vi "Simple TCP - Client.vi"() -> ()   [LabVIEW 2020]
doc: "Demonstrates how to open a connection to an TCP server, read the data being sent, and display the data on a chart. This VI is designed to stop if the TCP connection is terminated."
panel:
  out "Color Box":u32(colorbox)
  in  "Test Mode:":string(combo)
  in  "Stop":bool
  out "Status":string
  in  "Start":bool
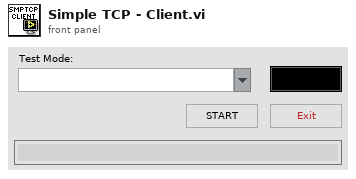
[diagram p1: front panel]
types:
  T1 = enum32{"Invalid", "Standard", "Closed", "Hidden", "Minimized", "Maximized"}
  T2 = enum32{"invalid app kind", "Development System", "Run Time System", "Student Edition", "Embedded LabVIEW", "Evaluation", "Custom"}
  T3 = cluster{"Core":cluster{"Current VI Reference":refnum<vi>, "Close Panel on Exit?":bool}, "Your Boolean data":bool, "IP Address":string, "port":u16, "connection ID":refnum<k5>, "Status":string, "Command":string, "Response":string}
  T4 = cluster{"Current VI Reference":refnum<vi>, "Close Panel on Exit?":bool}
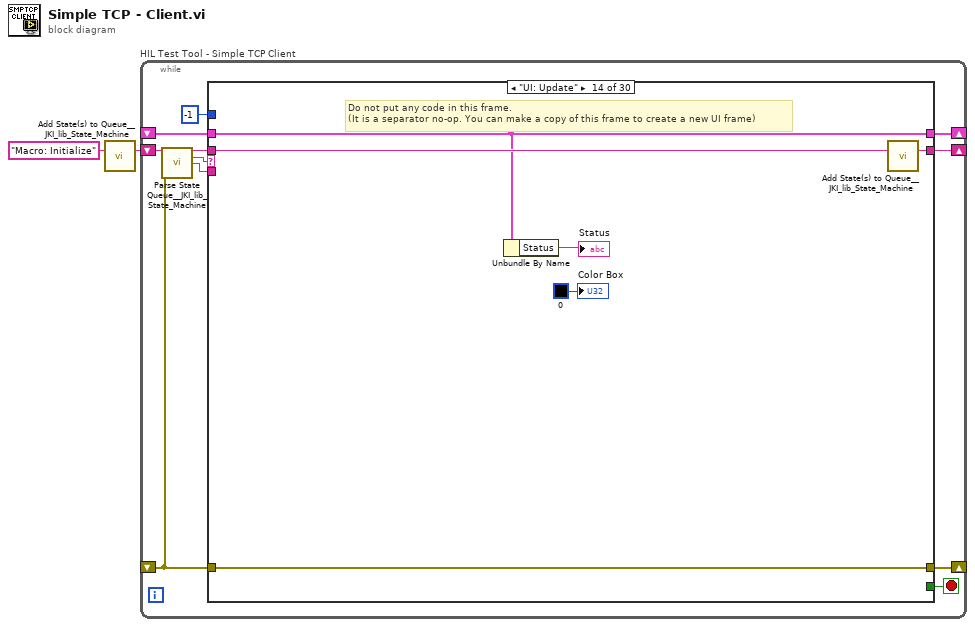
[diagram p0: block diagram]
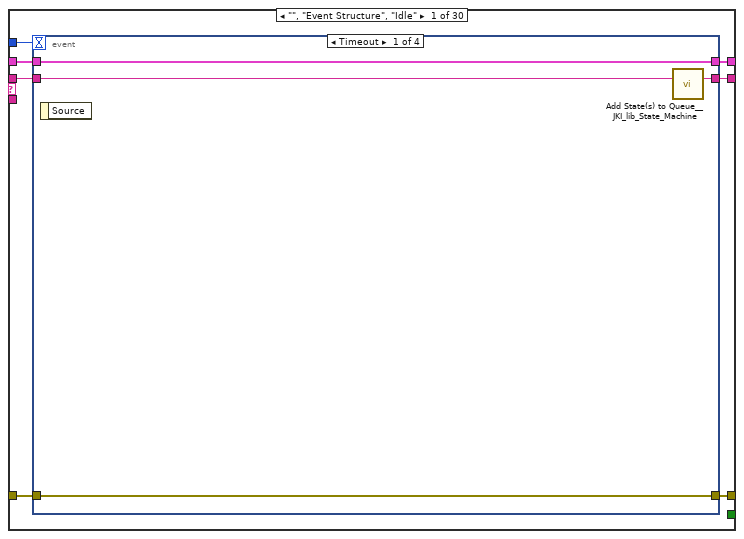
[diagram p2: hidden frame]
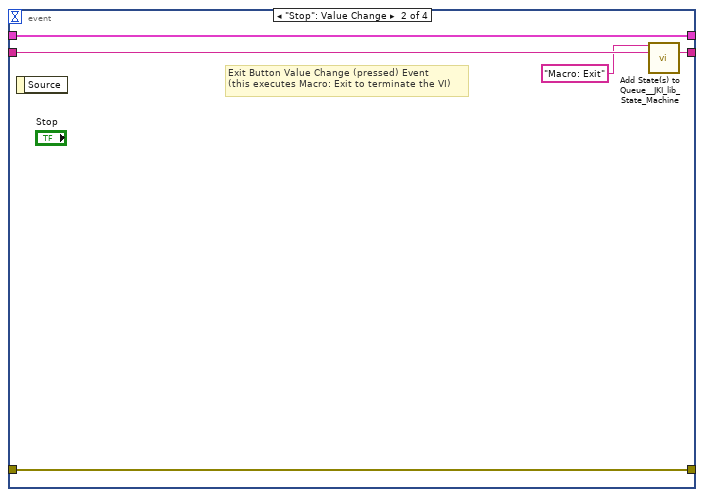
[diagram p3: hidden frame]
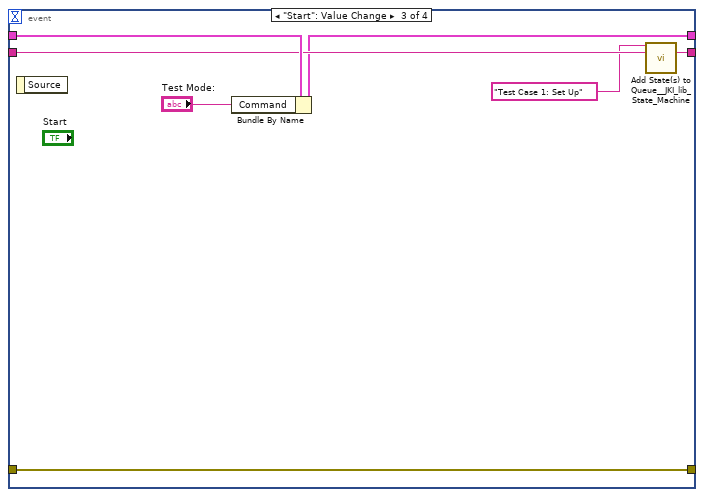
[diagram p4: hidden frame]
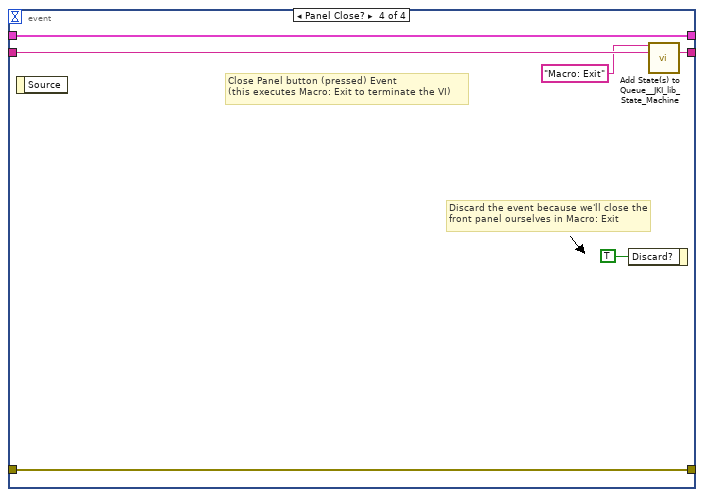
[diagram p5: hidden frame]
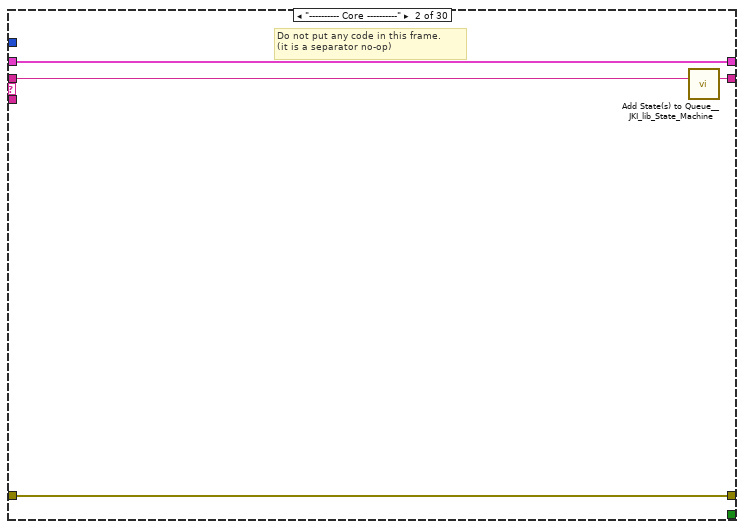
[diagram p6: hidden frame]
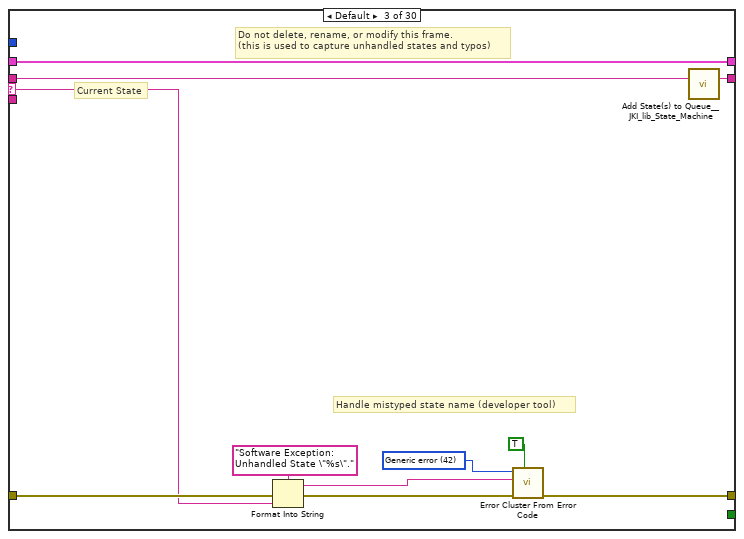
[diagram p7: hidden frame]
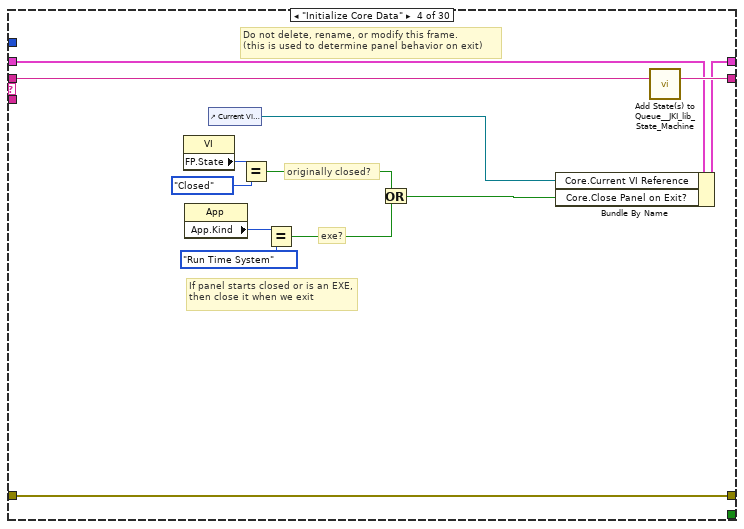
[diagram p8: hidden frame]
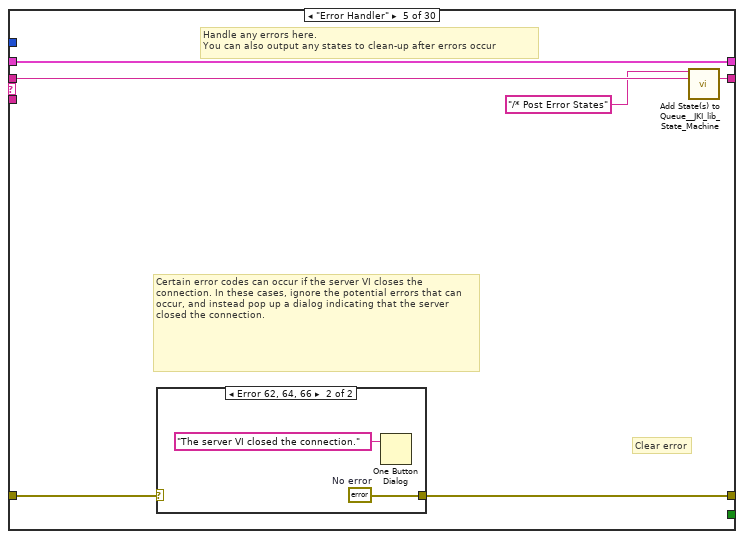
[diagram p9: hidden frame]
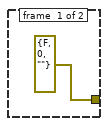
[diagram p10: hidden frame]
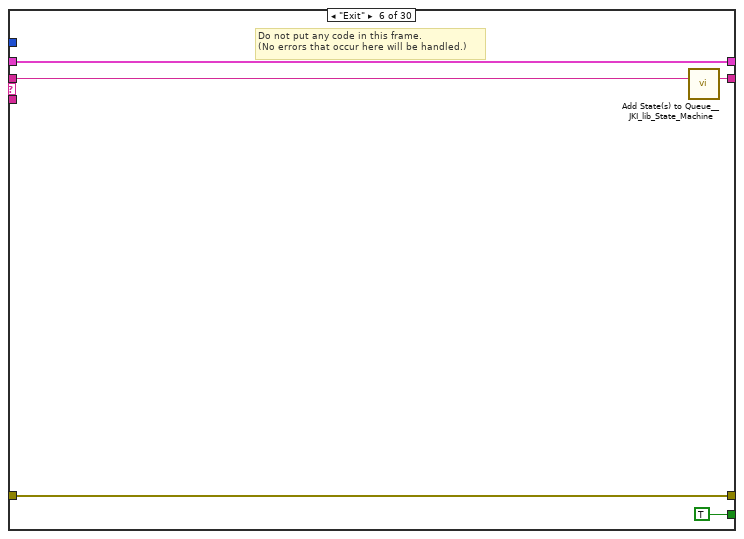
[diagram p11: hidden frame]
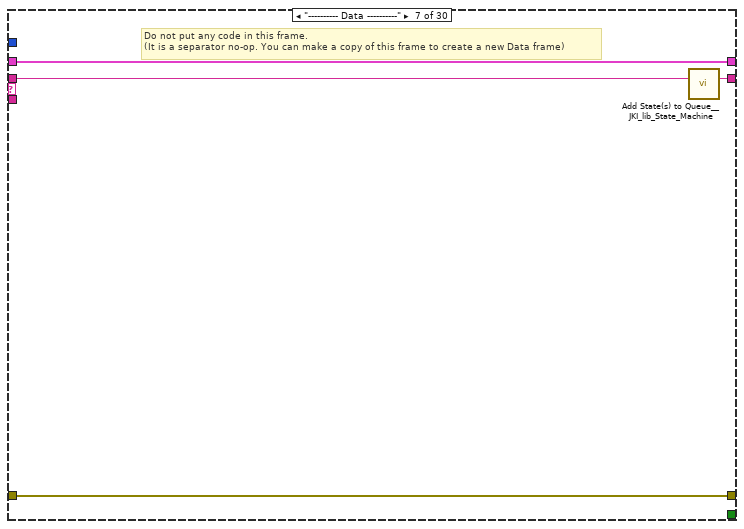
[diagram p12: hidden frame]
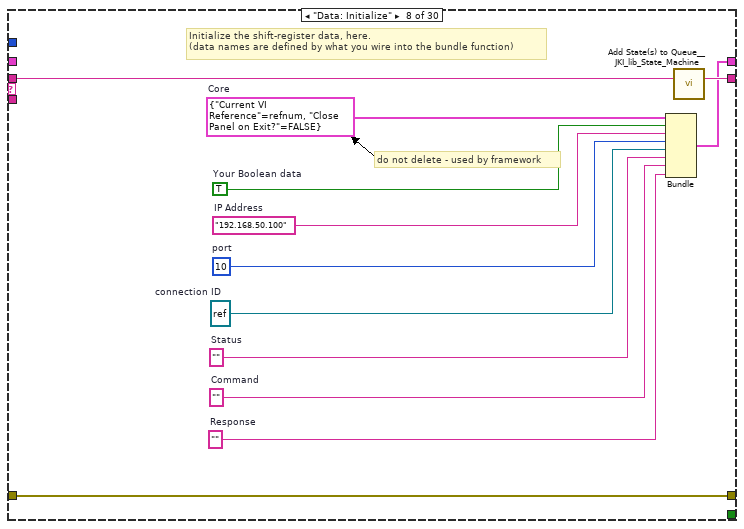
[diagram p13: hidden frame]
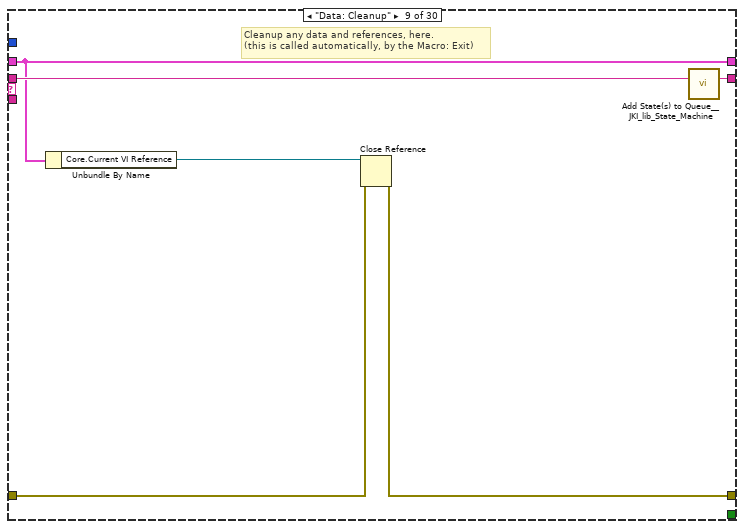
[diagram p14: hidden frame]
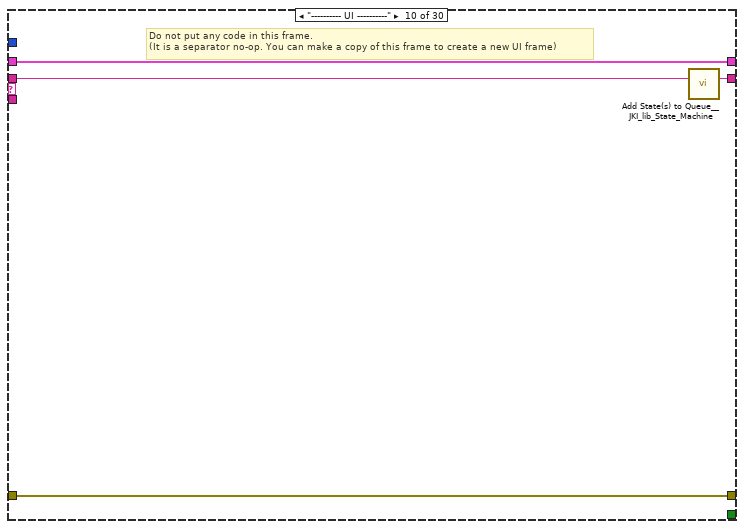
[diagram p15: hidden frame]
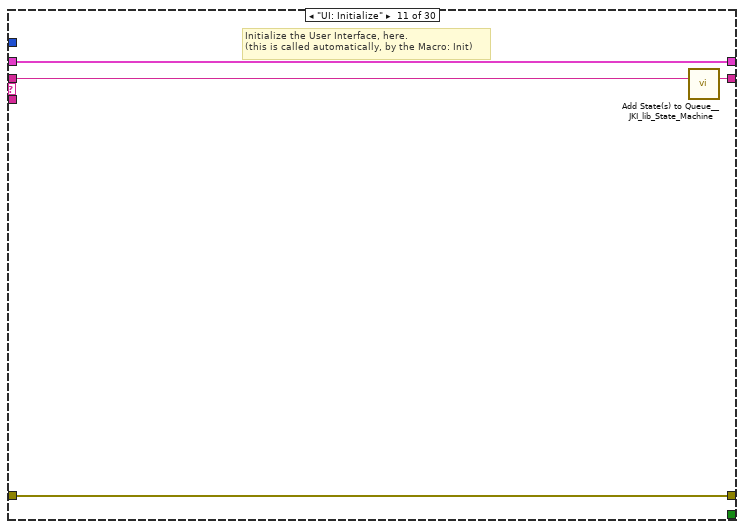
[diagram p16: hidden frame]
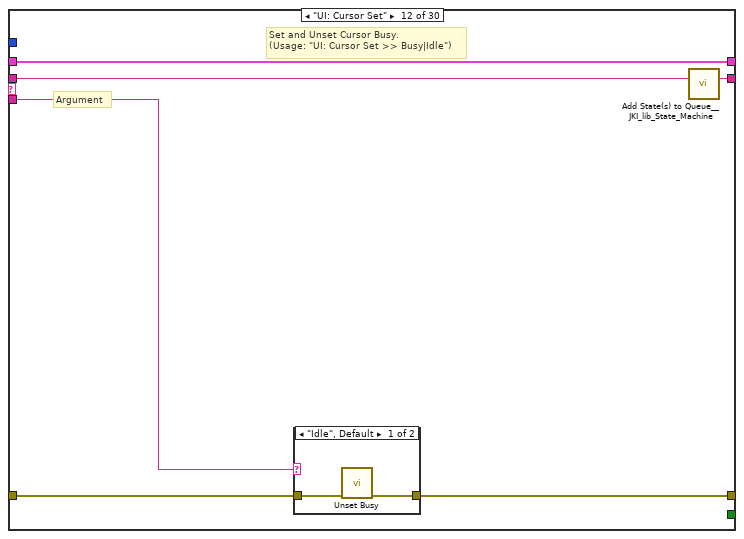
[diagram p17: hidden frame]
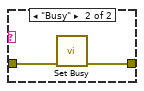
[diagram p18: hidden frame]
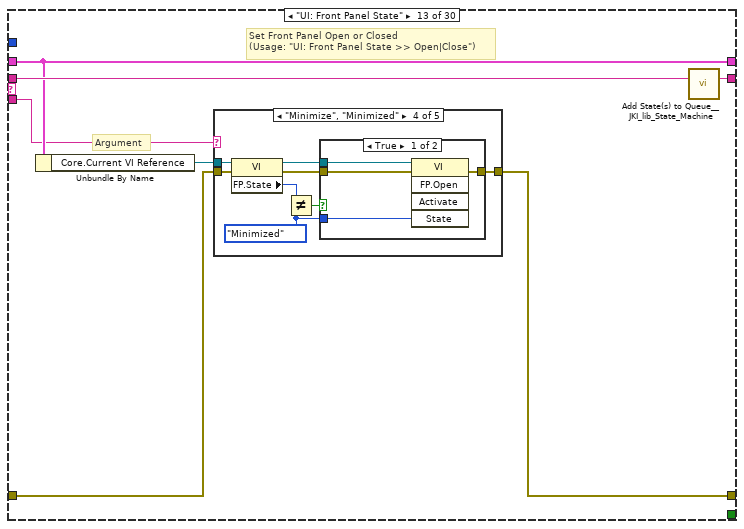
[diagram p19: hidden frame]
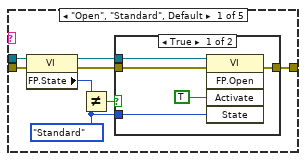
[diagram p20: hidden frame]
diagram:
  n1 = call <vilib>:"Add State(s) to Queue__JKI_lib_State_Machine.vi"("State(s) in (\"\")"="Macro: Initialize") -> ("States Out"=w2:string)  [unwired: 14 in]
  n2 = while "HIL Test Tool - Simple TCP Client" {
    shift-right: [w6] -> _
    shift-left: _ -> [w5]
    shift-right: [w9] -> _
    shift-left: _ -> [w3]
    shift-right: [w8] -> _
    shift-left: w2 -> [w10]
    stop <- w7 stop-if-true
    n3 = call <vilib>:"Parse State Queue__JKI_lib_State_Machine.vi"("State Queue"=w10, "Error In (no error)"=w3) -> ("Remaining States"=w12:string, "Current State"=w13:string, "Arguments"=w11:string)  [unwired: 11 in]
    n4 = case shown="\"UI: Update\"" w13 {
      selector: w13 -> [_ _ w47 _ _ _ _ _ _ _ _ _ _ _ _ _ _ _ _ _ _ _ _ _ _ _ _ _ _ _]
      tunnel: w12 -> [w20 w46 w51 w70 w76 w84 w88 w100 w106 w110 w114 w120 w131 w202 w206 w211 w216 w226 w230 w239 w247 w253 w257 w260 w266 w269 w273 w277 w283 w286]
      tunnel: w11 -> [_ _ _ _ _ _ _ _ _ _ _ w115 w125 _ _ _ _ _ _ _ _ _ _ _ _ _ _ _ _ _]
      tunnel: w5 -> [w18 w43 w49 w63 w74 w82 w85 _ w101 w107 w112 w118 w127 w199 w203 w208 w213 w223 w227 w237 w243 w249 w254 w258 w262 w267 w270 w274 w279 w284]
      tunnel: [w17 w44 w53 w67 w71 w81 w86 w97 w102 w108 w111 w116 w128 w200 w204 w209 w214 w224 w228 w233 w244 w250 w255 w259 w264 w268 w271 w275 w281 w285] -> w9
      tunnel: w3 -> [w16 w44 w52 w67 w72 w81 w86 w97 w103 w108 w111 w117 w129 w200 w204 w209 w214 w224 w228 w234 w245 w251 w255 w259 w265 w268 w271 w275 w282 w285]
      tunnel: [w19 w45 w50 w69 w75 w83 w87 w99 w105 w109 w113 w119 w130 w201 w205 w210 w215 w225 w229 w238 w246 w252 w256 w260 w266 w269 w272 w276 w283 w286] -> w8
      tunnel: [_ _ _ _ _ TRUE _ _ _ _ _ _ _ _ _ _ _ _ _ _ _ _ _ _ _ _ _ _ _ _] -> w7
      tunnel: [w15 w43 w49 w68 w74 w82 w85 w98 w101 w107 w112 w118 w127 w199 w203 w208 w213 w223 w227 w232 w241 w249 w254 w258 w262 w267 w270 w274 w279 w284] -> w6
      tunnel: -1 ("Timeout") -> [w14 _ _ _ _ _ _ _ _ _ _ _ _ _ _ _ _ _ _ _ _ _ _ _ _ _ _ _ _ _]
      frame "", "Event Structure", "Idle" {
        n5 = event shown="[0] Timeout" {
          selector: _ -> [_ _ _ _]
          dyn-events: _ -> [_ _ _ _]
          timeout: w14 -> [_ _ _ _]
          tunnel: w20 -> [w24 w29 w33 w42]
          tunnel: [w23 w28 w34 w41] -> w19
          tunnel: w18 -> [w22 w26 w36 w39]
          tunnel: [w21 w27 w35 w40] -> w17
          tunnel: w16 -> [w21 w27 w35 w40]
          tunnel: [w22 w26 w31 w39] -> w15
          event Timeout {
            n6 = event-data() -> ()  [unwired: 1 in, 1 out]
            n7 = call <vilib>:"Add State(s) to Queue__JKI_lib_State_Machine.vi"("State(s) in (\"\")"=w24) -> ("States Out"=w23:string)  [unwired: 14 in]
          }
          event "Stop": Value Change {
            # "Exit Button Value Change (pressed) Event\n(this executes Macro: Exit to terminate the VI)"
            n8 = event-data() -> ()  [unwired: 1 in, 1 out]
            n9 = call <vilib>:"Add State(s) to Queue__JKI_lib_State_Machine.vi"("State(s) in Front (\"\")"="Macro: Exit", "State(s) in (\"\")"=w29) -> ("States Out"=w28:string)  [unwired: 13 in]
          }
          event "Start": Value Change {
            n10 = event-data() -> ()  [unwired: 1 in, 1 out]
            n11 = Bundle By Name(cluster=w36, "Command"="Test Mode:") -> (w31:T3)
            n12 = call <vilib>:"Add State(s) to Queue__JKI_lib_State_Machine.vi"("State(s) in Front (\"\")"="Test Case 1: Set Up" ("State(s) in Front (\"\")"), "State(s) in (\"\")"=w33) -> ("States Out"=w34:string)  [unwired: 13 in]
          }
          event Panel Close? {
            # "Discard the event because we'll close the front panel ourselves in Macro: Exit"
            # "Close Panel button (pressed) Event\n(this executes Macro: Exit to terminate the VI)"
            n13 = event-data() -> ()  [unwired: 1 in, 1 out]
            n14 = event-data("Discard?"=TRUE) -> ()  [unwired: 1 in, 1 out]
            n15 = call <vilib>:"Add State(s) to Queue__JKI_lib_State_Machine.vi"("State(s) in Front (\"\")"="Macro: Exit", "State(s) in (\"\")"=w42) -> ("States Out"=w41:string)  [unwired: 13 in]
          }
        }
      }
      frame "---------- Core ----------" {
        # "Do not put any code in this frame.\n(it is a separator no-op)"
        n16 = call <vilib>:"Add State(s) to Queue__JKI_lib_State_Machine.vi"("State(s) in (\"\")"=w46) -> ("States Out"=w45:string)  [unwired: 14 in]
      }
      frame Default {
        w56 = 42 items=["No error", "Argument error", "Memory is full", "Out of zone", "End of file", "File already open", "Generic file I/O error", "File not found", "File permission error", "Disk is full", "Duplicate path", "Too many files open", "System feature not enabled", "Resource file not found", "Cannot add resource", "Resource not found", "Image not found", "Image memory error", "Pen does not exist", "Config type invalid", "Config token not found", "Config parse error", "Config memory error", "Bad external code format", "Bad external code offset", "External code not present", "Null window", "Destroy window error", "Null menu", "Print aborted", "Bad print record", "Print driver error", "Windows error during printing", "Memory error during printing", "Print dialog error", "Generic print error", "Invalid device refnum", "Device not found", "Device parameter error", "Device unit error", "Cannot open device", "Device call aborted", "Generic error", "Cancelled by user", "Object ID too low", "Object ID too high", "Object not in heap", "Unknown heap", "Unknown object (invalid DefProc)", "Unknown object (DefProc not in table)", "Message out of range", "Invalid (null) method", "Unknown message", "Manager call not supported", "Bad address", "Network operation in progress", "Network operation timed out", "Connection is busy", "Network attribute not supported", "Network error", "Address in use", "System out of memory", "Connection aborted", "Connection refused", "Not connected", "Already connected", "Connection closed", "Initialization error (interapplication manager)", "Bad occurrence", "Wait on unbound occurrence handler", "Occurrence queue overflow", "Datalog type conflict", "Unused", "Unrecognized type (interapplication manager)", "Memory corrupt", "Failed to make temporary DLL", "Old CIN version", "Drag socket not found", "Failed to load drop-object", "Failed to register OLE object", "Failed to release OLE object", "Format specifier type mismatch", "Unknown format specifier", "Too few format specifiers", "Too many format specifiers", "Scan failed", "Newer CIN version", "Error converting to variant", "Runtime menu error", "Password tampered", "Variant attribute not found", "Incompatible variant data type", "Event data is not available", "Event Store is not present", "Occurrence is not found", "Event Queue is not created", "Event info is not available", "Refnum passed is NULL", "Error retrieving Class GUID", "Error retrieving CoClass GUID", "Error retrieving TypeLib GUID.", "Bad built application magic bytes.", "Specific driver is different from the specific driver associated with the Logical Name.", "There is no session opened to the class driver.", "Max Error", "MAX - Error with config objects", "MAX - Error loading configuration", "MAX - Group not supported"]
        # "Current State"
        # "Do not delete, rename, or modify this frame.\n(this is used to capture unhandled states and typos)"
        # "Handle mistyped state name (developer tool)"
        n17 = Format Into String(format string="Software Exception: Unhandled State \"%s\"." ("message"), error in=w52, w47) -> (resulting string=w55:string, error out=w54:errorcluster)  [unwired: 1 in]
        n18 = call <vilib>:"Error Cluster From Error Code.vi"("show call chain? (False)"=TRUE, "error in (no error)"=w54, "error message (\"\")"=w55, "error code (0)"=w56) -> ("error out"=w53:errorcluster)  [unwired: 5 in]
        n19 = call <vilib>:"Add State(s) to Queue__JKI_lib_State_Machine.vi"("State(s) in (\"\")"=w51) -> ("States Out"=w50:string)  [unwired: 14 in]
      }
      frame "Initialize Core Data" {
        # "Do not delete, rename, or modify this frame.\n(this is used to determine panel behavior on exit)"
        # "originally closed?"
        # "exe?"
        # "If panel starts closed or is an EXE, then close it when we exit"
        n20 = property class="VI"() -> ("FP.State"=w60:T1)  [unwired: 2 in, 2 out]
        n21 = property class="App"() -> ("App.Kind"=w66:T2)  [unwired: 2 in, 2 out]
        n22 = control-ref of="Current VI Reference"() -> (w61:refnum<vi>)
        n23 = Equal?(x=w60, y=T1."Closed" ("Front Panel Window:State")) -> (x = y?=w58:bool)
        n24 = Equal?(x=w66, y=T2."Run Time System" ("Application:Kind")) -> (x = y?=w64:bool)
        n25 = Or(x=w58, y=w64) -> (x .or. y?=w62:bool)
        n26 = Bundle By Name(cluster=w63, "Core.Current VI Reference"=w61, "Core.Close Panel on Exit?"=w62) -> (w68:T3)
        n27 = call <vilib>:"Add State(s) to Queue__JKI_lib_State_Machine.vi"("State(s) in (\"\")"=w70) -> ("States Out"=w69:string)  [unwired: 14 in]
      }
      frame "Error Handler" {
        # "Certain error codes can occur if the server VI closes the connection. In these cases, ignore the potential errors that can occur, and instead pop up a dialog indicating that the server closed the connection."
        # "Handle any errors here.\nYou can also output any states to clean-up after errors occur"
        # "Clear error"
        n28 = case shown="Error 62, 64, 66" w72 {
          tunnel: [errorcluster {"status"=FALSE, "code"=0, "source"=""} ("No error") w79] -> w71
          frame #0 {
          }
          frame #1 {
            w79 = errorcluster {"status"=FALSE, "code"=0, "source"=""}  # No error
            n29 = One Button Dialog(message="The server VI closed the connection.") -> ()  [unwired: 1 in, 1 out]
          }
        }
        n30 = call <vilib>:"Add State(s) to Queue__JKI_lib_State_Machine.vi"("State(s) in Front (\"\")"="/* Post Error States", "State(s) in (\"\")"=w76) -> ("States Out"=w75:string)  [unwired: 13 in]
      }
      frame "Exit" {
        # "Do not put any code in this frame.\n(No errors that occur here will be handled.)"
        n31 = call <vilib>:"Add State(s) to Queue__JKI_lib_State_Machine.vi"("State(s) in (\"\")"=w84) -> ("States Out"=w83:string)  [unwired: 14 in]
      }
      frame "---------- Data ----------" {
        # "Do not put any code in this frame.\n(It is a separator no-op. You can make a copy of this frame to create a new Data frame)"
        n32 = call <vilib>:"Add State(s) to Queue__JKI_lib_State_Machine.vi"("State(s) in (\"\")"=w88) -> ("States Out"=w87:string)  [unwired: 14 in]
      }
      frame "Data: Initialize" {
        w89 = ""  # Response
        w90 = ""  # Command
        w91 = ""  # Status
        w92 = refnum<k5> refnum  # connection ID
        w93 = u16 10  # port
        w94 = T4 {"Current VI Reference"=refnum, "Close Panel on Exit?"=FALSE}  # Core
        w96 = TRUE  # Your Boolean data
        w95 = "192.168.50.100"  # IP Address
        # "do not delete - used by framework"
        # "Initialize the shift-register data, here.\n(data names are defined by what you wire into the bundle function)"
        n33 = Bundle("Core"=w94, "Your Boolean data"=w96, "IP Address"=w95, "port"=w93, "connection ID"=w92, "Status"=w91, "Command"=w90, "Response"=w89) -> (w98:T3)  [unwired: 1 in]
        n34 = call <vilib>:"Add State(s) to Queue__JKI_lib_State_Machine.vi"("State(s) in (\"\")"=w100) -> ("States Out"=w99:string)  [unwired: 14 in]
      }
      frame "Data: Cleanup" {
        # "Cleanup any data and references, here.\n(this is called automatically, by the Macro: Exit)"
        n35 = Unbundle By Name(w101) -> ("Core.Current VI Reference"=w104:refnum<vi>)
        n36 = Close Reference(reference=w104, error in (no error)=w103) -> (error out=w102:errorcluster)
        n37 = call <vilib>:"Add State(s) to Queue__JKI_lib_State_Machine.vi"("State(s) in (\"\")"=w106) -> ("States Out"=w105:string)  [unwired: 14 in]
      }
      frame "---------- UI ----------" {
        # "Do not put any code in this frame.\n(It is a separator no-op. You can make a copy of this frame to create a new UI frame)"
        n38 = call <vilib>:"Add State(s) to Queue__JKI_lib_State_Machine.vi"("State(s) in (\"\")"=w110) -> ("States Out"=w109:string)  [unwired: 14 in]
      }
      frame "UI: Initialize" {
        # "Initialize the User Interface, here.\n(this is called automatically, by the Macro: Init)"
        n39 = call <vilib>:"Add State(s) to Queue__JKI_lib_State_Machine.vi"("State(s) in (\"\")"=w114) -> ("States Out"=w113:string)  [unwired: 14 in]
      }
      frame "UI: Cursor Set" {
        # "Argument"
        # "Set and Unset Cursor Busy.\n(Usage: \"UI: Cursor Set >> Busy|Idle\")"
        n40 = case shown="\"Idle\", Default" w115 {
          tunnel: w117 -> [w122 w124]
          tunnel: [w121 w123] -> w116
          frame "Idle", Default {
            n41 = call <vilib>:"Unset Busy.vi"("error in (no error)"=w122) -> ("error out"=w121:errorcluster)  [unwired: 10 in]
          }
          frame "Busy" {
            n42 = call <vilib>:"Set Busy.vi"("error in (no error)"=w124) -> ("error out"=w123:errorcluster)  [unwired: 9 in, 1 out]
          }
        }
        n43 = call <vilib>:"Add State(s) to Queue__JKI_lib_State_Machine.vi"("State(s) in (\"\")"=w120) -> ("States Out"=w119:string)  [unwired: 14 in]
      }
      frame "UI: Front Panel State" {
        # "Argument"
        # "Set Front Panel Open or Closed\n(Usage: \"UI: Front Panel State >> Open|Close\")"
        n44 = Unbundle By Name(w127) -> ("Core.Current VI Reference"=w126:refnum<vi>)
        n45 = case shown="\"Minimize\", \"Minimized\"" w125 {
          tunnel: w129 -> [w137 w152 w163 w176 w189]
          tunnel: [w139 w153 w165 w178 w191] -> w128
          tunnel: w126 -> [w138 w150 w164 w177 w190]
          frame "Open", "Standard", Default {
            w132 = T1."Standard" ("State")
            n46 = property class="VI"(reference=w138, error in=w137) -> (reference out=w135:refnum<vi>, error out=w136:errorcluster, "FP.State"=w134:T1)
            n47 = Not Equal?(x=w134, y=w132) -> (x != y?=w133:bool)
            n48 = case shown="True" w133 {
              tunnel: [w143 w145] -> w139
              tunnel: w136 -> [w142 w145]
              tunnel: w135 -> [w141 _]
              tunnel: w132 -> [w140 _]
              frame True {
                n49 = invoke class="VI" method="FP.Open"(reference=w141, error in=w142, "Activate"=TRUE, "State"=w140) -> (error out=w143:errorcluster)  [unwired: 1 in, 4 out]
              }
              frame False {
              }
            }
          }
          frame "Close", "Closed" {
            n50 = property class="VI"(reference=w150, error in=w152) -> (reference out=w149:refnum<vi>, error out=w151:errorcluster, "FP.State"=w147:T1)
            n51 = Not Equal?(x=w147, y=T1."Closed" ("Front Panel Window:State")) -> (x != y?=w146:bool)
            n52 = case shown="True" w146 {
              tunnel: [w154 w157] -> w153
              tunnel: w151 -> [w154 w156]
              tunnel: w149 -> [_ w155]
              frame False {
              }
              frame True {
                n53 = invoke class="VI" method="FP.Close"(reference=w155, error in=w156) -> (error out=w157:errorcluster)  [unwired: 1 in, 2 out]
              }
            }
          }
          frame "Hidden", "Hide" {
            w158 = T1."Hidden" ("State")
            n54 = property class="VI"(reference=w164, error in=w163) -> (reference out=w161:refnum<vi>, error out=w162:errorcluster, "FP.State"=w160:T1)
            n55 = Not Equal?(x=w160, y=w158) -> (x != y?=w159:bool)
            n56 = case shown="True" w159 {
              tunnel: [w169 w170] -> w165
              tunnel: w162 -> [w168 w170]
              tunnel: w161 -> [w167 _]
              tunnel: w158 -> [w166 _]
              frame True {
                n57 = invoke class="VI" method="FP.Open"(reference=w167, error in=w168, "State"=w166) -> (error out=w169:errorcluster)  [unwired: 2 in, 4 out]
              }
              frame False {
              }
            }
          }
          frame "Minimize", "Minimized" {
            w171 = T1."Minimized" ("State")
            n58 = property class="VI"(reference=w177, error in=w176) -> (reference out=w174:refnum<vi>, error out=w175:errorcluster, "FP.State"=w173:T1)
            n59 = Not Equal?(x=w173, y=w171) -> (x != y?=w172:bool)
            n60 = case shown="True" w172 {
              tunnel: [w182 w183] -> w178
              tunnel: w175 -> [w181 w183]
              tunnel: w174 -> [w180 _]
              tunnel: w171 -> [w179 _]
              frame True {
                n61 = invoke class="VI" method="FP.Open"(reference=w180, error in=w181, "State"=w179) -> (error out=w182:errorcluster)  [unwired: 2 in, 4 out]
              }
              frame False {
              }
            }
          }
          frame "Maximize", "Maximized" {
            w184 = T1."Maximized" ("State")
            n62 = property class="VI"(reference=w190, error in=w189) -> (reference out=w187:refnum<vi>, error out=w188:errorcluster, "FP.State"=w186:T1)
            n63 = Not Equal?(x=w186, y=w184) -> (x != y?=w185:bool)
            n64 = case shown="True" w185 {
              tunnel: [w195 w196] -> w191
              tunnel: w188 -> [w194 w196]
              tunnel: w187 -> [w193 _]
              tunnel: w184 -> [w192 _]
              frame True {
                n65 = invoke class="VI" method="FP.Open"(reference=w193, error in=w194, "State"=w192) -> (error out=w195:errorcluster)  [unwired: 2 in, 4 out]
              }
              frame False {
              }
            }
          }
        }
        n66 = call <vilib>:"Add State(s) to Queue__JKI_lib_State_Machine.vi"("State(s) in (\"\")"=w131) -> ("States Out"=w130:string)  [unwired: 14 in]
      }
      frame "UI: Update" {
        # "Do not put any code in this frame.\n(It is a separator no-op. You can make a copy of this frame to create a new UI frame)"
        n67 = Unbundle By Name(w199) -> ("Status"=→"Status":string)
        n68 = call <vilib>:"Add State(s) to Queue__JKI_lib_State_Machine.vi"("State(s) in (\"\")"=w202) -> ("States Out"=w201:string)  [unwired: 14 in]
        "Color Box" <- u32 0
      }
      frame "---------- Macro ----------" {
        # "Do not put any code in this frame.\n(It is a separator no-op. You can make a copy of this frame to create a new Macro frame)"
        n69 = call <vilib>:"Add State(s) to Queue__JKI_lib_State_Machine.vi"("State(s) in (\"\")"=w206) -> ("States Out"=w205:string)  [unwired: 14 in]
      }
      frame "Macro: Initialize" {
        w207 = "Data: Initialize\nInitialize Core Data\nUI: Initialize\nUI: Front Panel State >> Open"  # Data: Initialize Initialize Core Data UI: Initialize UI: Front Panel State >> Open
        # "Initialization Macro\n(This is called once, when the VI starts)"
        n70 = call <vilib>:"Add State(s) to Queue__JKI_lib_State_Machine.vi"("State(s) in Front (\"\")"=w207, "State(s) in (\"\")"=w211) -> ("States Out"=w210:string)  [unwired: 13 in]
      }
      frame "Macro: Test Case 1" {
        # "Do not put any code in this frame.\n(It is a separator no-op. You can make a copy of this frame to create a new Macro frame)"
        n71 = call <vilib>:"Add State(s) to Queue__JKI_lib_State_Machine.vi"("State(s) in Front (\"\")"="Test Case 1: MAIN\nTCP: Response\nUI: Update" ("State(s) in Front (\"\")"), "State(s) in (\"\")"=w216) -> ("States Out"=w215:string)  [unwired: 13 in]
      }
      frame "Macro: Exit" {
        # "Exit Macro\n(This is called once, when the VI exits)"
        n72 = Unbundle By Name(w223) -> ("Core.Close Panel on Exit?"=w222:bool)
        n73 = Select(t="UI: Front Panel State >> Close", s=w222, f="") -> (s? t:f=w219:string)
        n74 = call <vilib>:"Add State(s) to Queue__JKI_lib_State_Machine.vi"("State(s) in (\"\")"=w219, "State(s) at Back (\"\")"="Data: Cleanup\nExit") -> ("States Out"=w217:string)  [unwired: 13 in]
        n75 = call <vilib>:"Add State(s) to Queue__JKI_lib_State_Machine.vi"("State(s) in Front (\"\")"=w217, "State(s) in (\"\")"=w226) -> ("States Out"=w225:string)  [unwired: 13 in]
      }
      frame "---------- TCP ----------" {
        # "Template Separator\n(You can make a copy of, or modify, this frame)"
        n76 = call <vilib>:"Add State(s) to Queue__JKI_lib_State_Machine.vi"("State(s) in (\"\")"=w230) -> ("States Out"=w229:string)  [unwired: 14 in]
      }
      frame "TCP: Open Connection" {
        # "Open a TCP connection with the TCP Open Connection function."
        # "Do not put any code in this frame.\n(it is a separator no-op)"
        n77 = Unbundle By Name(w237) -> ("IP Address"=w236:string, "port"=w235:u16)
        n78 = TCP Open Connection(address=w236, remote port or service name=w235, error in (no error)=w234) -> (connection ID=w231:refnum<k5>, error out=w233:errorcluster)  [unwired: 2 in]
        n79 = Bundle By Name(cluster=w237, "connection ID"=w231) -> (w232:T3)
        n80 = call <vilib>:"Add State(s) to Queue__JKI_lib_State_Machine.vi"("State(s) in (\"\")"=w239) -> ("States Out"=w238:string)  [unwired: 14 in]
      }
      frame "TCP: Response" {
        # "Template Separator\n(You can make a copy of, or modify, this frame)"
        n81 = Unbundle By Name(w243) -> ("connection ID"=w242:refnum<k5>)
        n82 = TCP Read(connection ID=w242, error in (no error)=w245) -> (data out=w240:string, error out=w244:errorcluster)  [unwired: 3 in, 1 out]
        n83 = Bundle By Name(cluster=w243, "Response"=w240) -> (w241:T3)
        n84 = call <vilib>:"Add State(s) to Queue__JKI_lib_State_Machine.vi"("State(s) in (\"\")"=w247) -> ("States Out"=w246:string)  [unwired: 14 in]
      }
      frame "TCP: Close Connection" {
        # "TCP Close Connection closes the connection when the user clicks Stop or an error occurs."
        # "Do not put any code in this frame.\n(it is a separator no-op)"
        n85 = Unbundle By Name(w249) -> ("connection ID"=w248:refnum<k5>)
        n86 = TCP Close Connection(connection ID=w248, error in (no error)=w251) -> (error out=w250:errorcluster)  [unwired: 1 in, 1 out]
        n87 = call <vilib>:"Add State(s) to Queue__JKI_lib_State_Machine.vi"("State(s) in (\"\")"=w253) -> ("States Out"=w252:string)  [unwired: 14 in]
      }
      frame "---------- Test Case 1 ----------" {
        # "Template Separator\n(You can make a copy of, or modify, this frame)"
        n88 = call <vilib>:"Add State(s) to Queue__JKI_lib_State_Machine.vi"("State(s) in (\"\")"=w257) -> ("States Out"=w256:string)  [unwired: 14 in]
      }
      frame "Test Case 1: Set Up" {
        # "Template Separator\n(You can make a copy of, or modify, this frame)"
      }
      frame "Test Case 1: MAIN" {
        # "Your code here.\n(You can make a copy of, or modify, this frame)"
        n89 = Unbundle By Name(w262) -> ("connection ID"=w263:refnum<k5>)
        n90 = TCP Write(connection ID=w263, data in="Test1", error in (no error)=w265) -> (error out=w264:errorcluster)  [unwired: 1 in, 2 out]
      }
      frame "Test Case 1: Clean Up" {
        # "Template Separator\n(You can make a copy of, or modify, this frame)"
      }
      frame "---------- Test Case 2 ----------" {
        # "Template Separator\n(You can make a copy of, or modify, this frame)"
        n91 = call <vilib>:"Add State(s) to Queue__JKI_lib_State_Machine.vi"("State(s) in (\"\")"=w273) -> ("States Out"=w272:string)  [unwired: 14 in]
      }
      frame "Test Case 2: Set Up" {
        # "Template Separator\n(You can make a copy of, or modify, this frame)"
        n92 = call <vilib>:"Add State(s) to Queue__JKI_lib_State_Machine.vi"("State(s) in (\"\")"=w277) -> ("States Out"=w276:string)  [unwired: 14 in]
      }
      frame "Test Case 2: MAIN" {
        # "Your code here.\n(You can make a copy of, or modify, this frame)"
        n93 = Unbundle By Name(w279) -> ("connection ID"=w280:refnum<k5>)
        n94 = TCP Write(connection ID=w280, data in="Test2", error in (no error)=w282) -> (error out=w281:errorcluster)  [unwired: 1 in, 2 out]
      }
      frame "Test Case 2: Clean Up" {
        # "Template Separator\n(You can make a copy of, or modify, this frame)"
      }
    }
  }
